vi "get runtime class name.vi"(8 "error in":errorcluster, 11 "CVT configuration in":refnum<class "testmod configuration.lvclass">) -> (0 "error out":errorcluster, 2 "class name":string, 3 "CVT configuration out":refnum<class "testmod configuration.lvclass">)   [LabVIEW 2013, in "testmod configuration.lvclass"]
doc: "Provides an interface for determining the module runtime class associated with this module configuration. This class name can then be used to dynamically load or locate the runtime class for initialization purposes."
uses:
  testmod configuration.lvclass
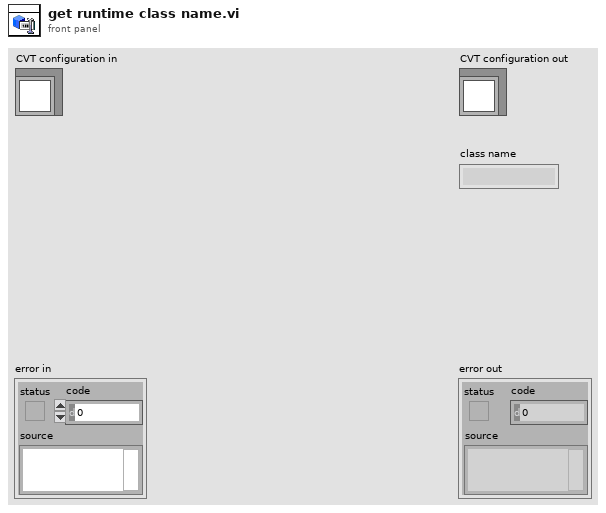
[diagram p1: front panel]
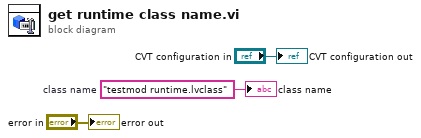
[diagram p0: block diagram]
diagram:
  w1 = "testmod runtime.lvclass"  # class name
  "error out" <- "error in"
  "CVT configuration out" <- "CVT configuration in"
  "class name" <- w1
